vi "Initconfiguration.vi"(8 "Error In":errorcluster) -> (0 "Error Out":errorcluster, 3 "Serial configuration":T1={"Serial Resource"="COM5", "data bits (8)"=8, "parity (0:none)"=enum."None", "flow control (0:none)"=0, "stop bits (10: 1 bit)"=10, "baud rate (9600)"=38400})   [LabVIEW 2010]
panel:
  in  "OK Button":bool
  in  "flow control (0:none)":u16(ring) items=["None", "XON/XOFF", "RTS/CTS", "XON/XOFF & RTS/CTS", "DTR/DSR", "XON/XOFF & DTR/DSR"]
  in  "stop bits (10: 1 bit)":u16(ring)=10 items=["1.0"=10, "1.5"=15, "2.0"=20]
  in  "parity (0:none)":enum16{"None", "Odd", "Even", "Mark", "Space"}(ring)
  in  "data bits (8)":u16=8 min=5 max=8 step=1
  in  "baud rate (9600)":u32=38400
  in  "Serial Resource":refnum<visa-resource-name>="COM5"
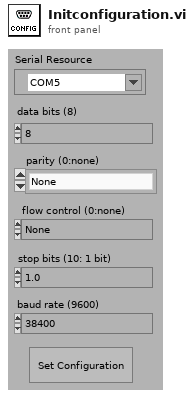
[diagram p1: front panel]
types:
  T1 = cluster{"Serial Resource":refnum<visa-resource-name>, "data bits (8)":u16, "parity (0:none)":enum16{"None", "Odd", "Even", "Mark", "Space"}, "flow control (0:none)":u16, "stop bits (10: 1 bit)":u16, "baud rate (9600)":u32}
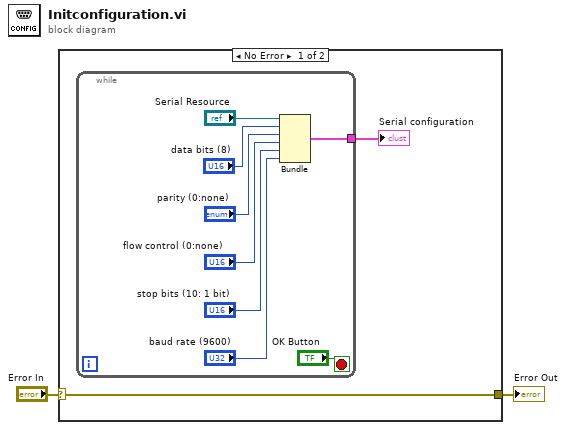
[diagram p0: block diagram]
diagram:
  n1 = case shown="No Error" "Error In" {
    selector: "Error In" -> [w3 w13]
    tunnel: [w3 w13] -> w1
    frame No Error {
      n2 = while {
        tunnel: [w5] -> w4
        stop <- "OK Button" stop-if-true
        n3 = Bundle("Serial Resource"="Serial Resource", "data bits (8)"="data bits (8)", "parity (0:none)"="parity (0:none)", "flow control (0:none)"="flow control (0:none)", "stop bits (10: 1 bit)"="stop bits (10: 1 bit)", "baud rate (9600)"="baud rate (9600)") -> (w5:T1)  [unwired: 1 in]
      }
      "Serial configuration" <- w4
    }
    frame Error {
    }
  }
  "Error Out" <- w1
